vi "SGL to IEEE754 Integer.vi"(10 "Number":sgl=-101.101 format="%.12f") -> (2 "IEEE754 INTEGER":fxp<+,32,32>)   [LabVIEW 2010]
panel:
  out "Sign":bool=TRUE
  out "Mantissa":bool[](array[boolean])=[TRUE, FALSE, FALSE, TRUE, FALSE, TRUE, FALSE, FALSE, FALSE, TRUE, TRUE, FALSE, FALSE, TRUE, TRUE, TRUE, FALSE, TRUE, TRUE, FALSE, TRUE, TRUE, FALSE]
  out "Exponent":bool[](array[boolean])=[TRUE, FALSE, FALSE, FALSE, FALSE, TRUE, FALSE, TRUE]
  out "Exponent":sgl=6.0 format="%.2f"
  out "Mantissa":sgl=1.5797031 format="%.8f"
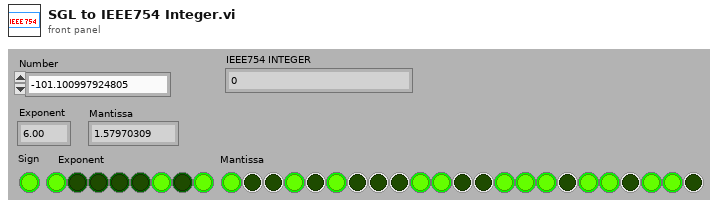
[diagram p1: front panel]
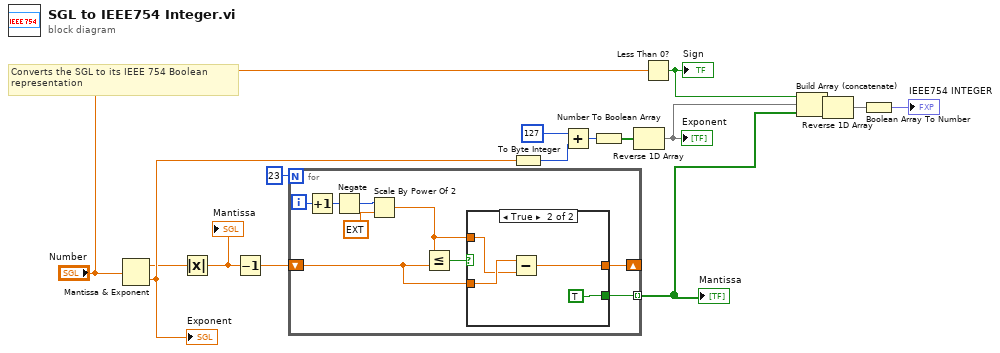
[diagram p0: block diagram]
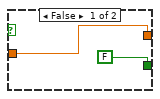
[diagram p2: hidden frame]
diagram:
  # "Converts the SGL to its IEEE 754 Boolean \nrepresentation"
  n1 = Mantissa & Exponent(0:"Number") -> (1:w7:sgl, 2:w10:sgl)
  "Exponent" <- w10
  n2 = Absolute Value(x=w7) -> (abs(x)=w8:sgl)
  "Mantissa" <- w8
  n3 = Decrement(x=w8) -> (x-1=w12:sgl)
  n4 = for {
    N: 23 -> [_]
    shift-right: [w18] -> _
    shift-left: w12 -> [w20]
    tunnel: [w17] -> w4 mode=indexing
    i -> [w25]
    n5 = Increment(x=w25) -> (x+1=w24:i32)
    n6 = Negate(x=w24) -> (-x=w23:i32)
    n7 = Scale By Power Of 2(n=w23, x=ext 1.0) -> (x*2^n=w19:ext)
    n8 = Less Or Equal?(x=w19, y=w20) -> (x <= y?=w21:bool)
    n9 = case shown="True" w21 {
      tunnel: w20 -> [w26 w31]
      tunnel: w19 -> [_ w28]
      tunnel: [w26 w30] -> w18
      tunnel: [FALSE TRUE] -> w17
      frame False {
      }
      frame True {
        n10 = Subtract(x=w31, y=w28) -> (x-y=w30:ext)
      }
    }
  }
  "Mantissa" <- w4
  n11 = To Byte Integer(number=w10) -> (8bit integer=w16:i8)
  n12 = Add(x=i8 127, y=w16) -> (x+y=w15:i8)
  n13 = Number To Boolean Array(number=w15) -> (Boolean array=w14:bool[])
  n14 = Reverse 1D Array(array=w14) -> (reversed array=w5:bool[])
  "Exponent" <- w5
  n15 = Less Than 0?(x="Number") -> (x < 0?=w6:bool)
  "Sign" <- w6
  n16 = Build Array (concatenate)(w6, w5, w4) -> (w3:bool[])
  n17 = Reverse 1D Array(array=w3) -> (reversed array=w1:bool[])
  n18 = Boolean Array To Number(Boolean array=w1) -> (number=→"IEEE754 INTEGER":fxp<+,32,32>)
